vi "Apply Config.vi"(8 "Error In":errorcluster, 10 "Session Handle":refnum<k15>, 11 "object in":refnum<class "DC Config.lvclass">) -> (0 "Error Out":errorcluster, 3 "object out":refnum<class "DC Config.lvclass">)   [LabVIEW 2023, in "HAL.lvlib" / "PXI-5441.lvlib" / "DC Config.lvclass"]
uses:
  DC Config.lvclass
  DC Config.lvclass/DC Config.ctl
  <instrlib>/niFgen/niFgen.llb/niFgen Waveform Type.ctl
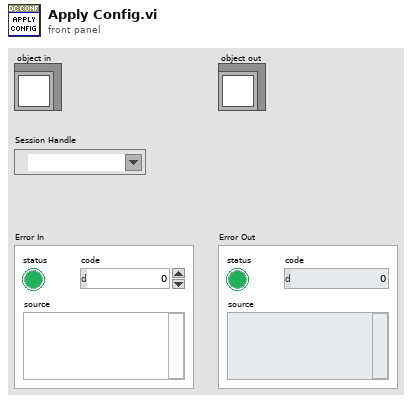
[diagram p1: front panel]
types:
  T1 = typedef "niFgen Waveform Type.ctl" = i32
  T2 = typedef "niFgen_ctl Exported Signal Desination Values (ComboBox).ctl" = string
  T3 = typedef "niFgen_ctl Exported Signal Name Values (Ring).ctl" = u16
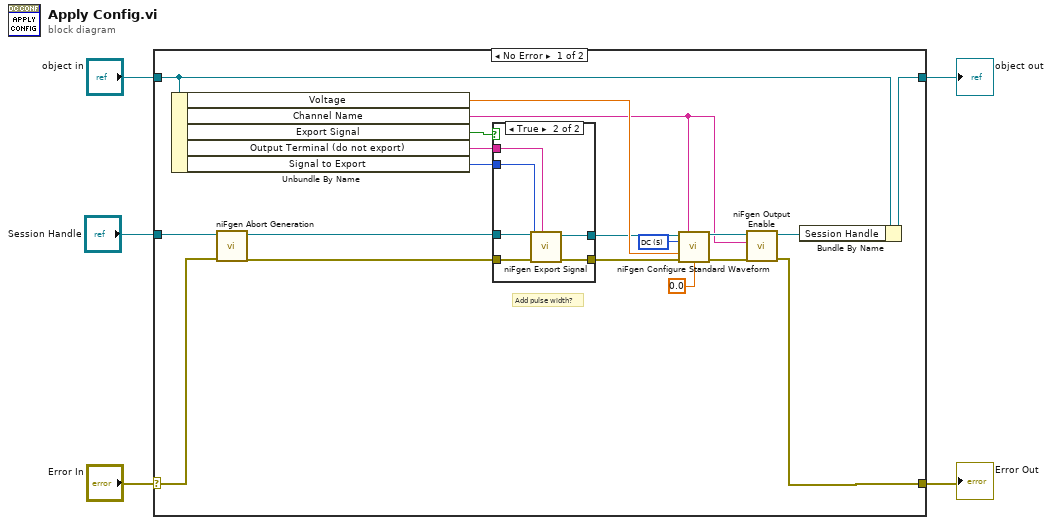
[diagram p0: block diagram]
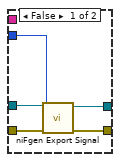
[diagram p2: hidden frame]
diagram:
  n1 = case shown="No Error" "Error In" {
    selector: "Error In" -> [w24 w37]
    tunnel: [w9 w37] -> w4
    tunnel: [w22 w36] -> w2
    tunnel: "object in" -> [w23 w36]
    tunnel: "Session Handle" -> [w17 _]
    frame No Error {
      w20 = T1 5 items=["Sine", "Square", "Triangle", "Ramp Up", "Ramp Down", "DC", "Noise", "User"] ("Waveform")
      # "Add pulse width?"
      n2 = Unbundle By Name(w23) -> ("Voltage"=w19:dbl, "Channel Name"=w6:string, "Export Signal"=w12:bool, "Output Terminal (do not export)"=w11:T2, "Signal to Export"=w10:T3)
      n3 = call <instrlib>:"niFgen Abort Generation.vi"("error in (no error)"=w24, "Instrument Handle"=w17) -> ("error out"=w18:errorcluster, "Instrument Handle Out"=w15:refnum<k15>)  [unwired: 8 in]
      n4 = case shown="True" w12 {
        tunnel: w18 -> [w29 w35]
        tunnel: [w28 w34] -> w16
        tunnel: w15 -> [w27 w33]
        tunnel: [w26 w32] -> w14
        tunnel: w11 -> [_ w31]
        tunnel: w10 -> [w25 w30]
        frame False {
          n5 = call <instrlib>:"niFgen Export Signal.vi"("error in (no error)"=w29, "Signal"=w25, "Instrument Handle"=w27) -> ("error out"=w28:errorcluster, "Instrument Handle Out"=w26:refnum<k15>)  [unwired: 7 in]
        }
        frame True {
          n6 = call <instrlib>:"niFgen Export Signal.vi"("Output Terminal (do not export)"=w31, "error in (no error)"=w35, "Signal"=w30, "Instrument Handle"=w33) -> ("error out"=w34:errorcluster, "Instrument Handle Out"=w32:refnum<k15>)  [unwired: 6 in]
        }
      }
      n7 = call <instrlib>:"niFgen Configure Standard Waveform.vi"("Instrument Handle"=w14, "Channel Name"=w6, "Waveform"=w20, "Amplitude"=w19, "error in (no error)"=w16, "DC Offset"=0.0) -> ("Instrument Handle Out"=w8:refnum<k15>, "error out"=w21:errorcluster)  [unwired: 8 in]
      n8 = call <instrlib>:"niFgen Output Enable.vi"("error in (no error)"=w21, "Channel Name"=w6, "Instrument Handle"=w8) -> ("error out"=w9:errorcluster, "Instrument Handle Out"=w7:refnum<k15>)  [unwired: 7 in]
      n9 = Bundle By Name(cluster=w23, "Session Handle"=w7) -> (w22:refnum<class "DC Config.lvclass">)
    }
    frame Error {
    }
  }
  "Error Out" <- w4
  "object out" <- w2
